vi "TimeTaskerVr3.vi"(0 "Delay(sec)":dbl, 1 "Start Counting?":bool) -> (2 "TimePast?":bool, 3 "TimePast":dbl, 4 "Counting?":bool)   [LabVIEW 2012]
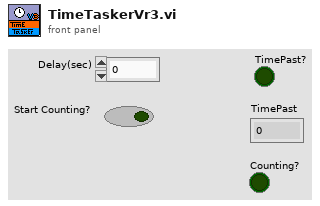
[diagram p1: front panel]
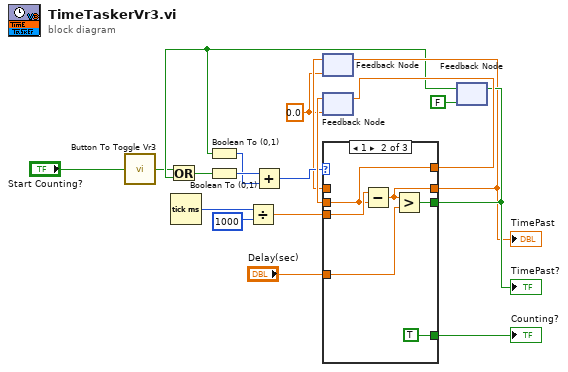
[diagram p0: block diagram]
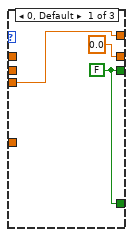
[diagram p2: hidden frame]
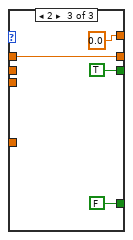
[diagram p3: hidden frame]
diagram:
  w5 = 0.0 ("f")
  n1 = call "Button To Toggle Vr3.vi"("InValue"="Start Counting?") -> ("Result"=w2:bool)
  n2 = Tick Count (ms)() -> (millisecond timer value=w18:u32)
  n3 = Divide(x=w18, y=u32 1000) -> (x/y=w16:dbl)
  n4 = feedback #1(w5) -> (w8:dbl)
  n5 = feedback #2(w5) -> (w14:dbl)
  n6 = feedback #3(FALSE ("Counting?")) -> (w4:bool)
  n7 = Or(x=w2, y=w4) -> (x .or. y?=w3:bool)
  n8 = Boolean To (0,1)(Boolean=w4) -> (0, 1=w9:i16)
  n9 = Boolean To (0,1)(Boolean=w3) -> (0, 1=w11:i16)
  n10 = Add(x=w11, y=w9) -> (x+y=w10:i16)
  n11 = case shown="1" w10 {
    tunnel: [0.0 w25 w31] -> w7
    tunnel: [w22 w23 TRUE ("Counting?")] -> w12
    tunnel: [w22 TRUE ("Counting?") FALSE ("Counting?")] -> w17
    tunnel: w16 -> [w20 w27 _]
    tunnel: [w20 w26 0.0 ("f")] -> w15
    tunnel: w14 -> [_ w26 _]
    tunnel: "Delay(sec)" -> [_ w24 _]
    tunnel: w8 -> [_ _ w31]
    frame 0, Default {
      w22 = FALSE ("Counting?")
    }
    frame 1 {
      n12 = Subtract(x=w27, y=w26) -> (x-y=w25:dbl)
      n13 = Greater?(x=w25, y=w24) -> (0:w23:bool)
    }
    frame 2 {
    }
  }
  "TimePast?" <- w12
  "Counting?" <- w17
  "TimePast" <- w7
  n14 = feedback-in #1(w7) -> ()
  n15 = feedback-in #2(w15) -> ()
  n16 = feedback-in #3(w12) -> ()
